vi "read_FWM_txt_file.vi"(11 "File path":path) -> (1 "Delay positiion":dbl[](array[numeric]), 2 "Wavelength":dbl[](array[numeric]), 3 "Intensity Graph":dbl[][](graph), 5 "File Name":path)   [LabVIEW 2009]
doc: "This Vi loads the FWM spreadsheet(.txt) file which is saved using AD-Spectroscopy-v2.2.vi"
uses:
  <vilib>/Utility/file.llb/Read From Spreadsheet File (DBL).vi
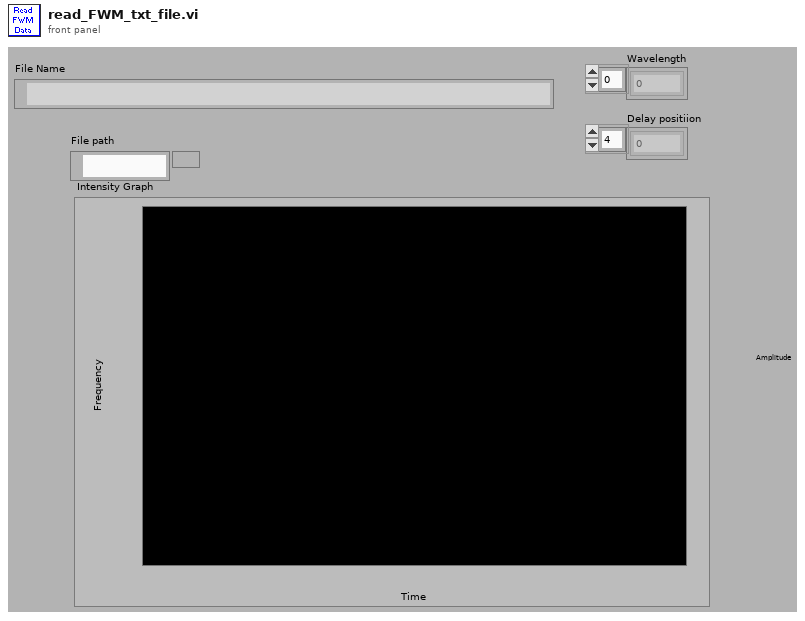
[diagram p1: front panel]
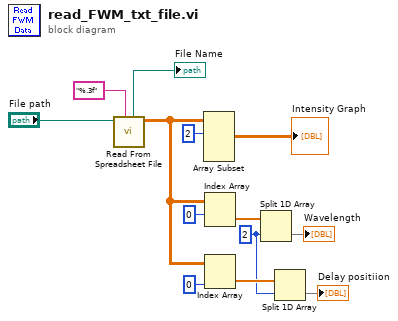
[diagram p0: block diagram]
diagram:
  w4 = 2 ("index")
  n1 = call-poly <vilib>:"Read From Spreadsheet File.vi"("format (%.3f)"="%.3f", "file path (dialog if empty)"="File path") -> ("all rows"=w7:dbl[][], "new file path (Not A Path if cancelled)"=→"File Name":path)  [unwired: 5 in, 3 out]
  n2 = Array Subset(array=w7, index (row)=2 ("index")) -> (→"Intensity Graph":dbl[][])  [unwired: 3 in]
  n3 = Index Array(array=w7, index (row)=0) -> (element=w9:dbl[])  [unwired: 1 in]
  n4 = Index Array(array=w7, index (col)=0 ("disabled index (col)")) -> (element=w5:dbl[])  [unwired: 1 in]
  n5 = Split 1D Array(array=w9, index=w4) -> (second subarray=→"Wavelength":dbl[])  [unwired: 1 out]
  n6 = Split 1D Array(array=w5, index=w4) -> (second subarray=→"Delay positiion":dbl[])  [unwired: 1 out]
